vi "NI 5772 (AC) - DigitizerFIFOAvg (FPGA).vi"() -> ()   [LabVIEW 2020]
doc: "Example Description:\nThis example demonstrates how to enable Time Interleaved Sampling with the NI 5772 adapter module to achieve a sampling rate of 1.6GS/s. This example continuously acquires records of analog input data from the NI 5772 adapter module. It allows you to select an AI channel, trigger type, and record size. This VI must be compiled before it is run. \n\nRunning the VI:\nThis VI must be run from the NI 5772 - Getting Started (Host).vi. Refer to the host VI documentation for steps regarding running and configuring the FPGA VI. \n\nExecution Steps:\nRefer to the Block Diagram of this VI for execution comments."
uses:
  Controls/AI Trigger Type.ctl
  Controls/Aquire State.ctl
  <vilib>/Platform/TimedLoop/XDataNode/timing_clust.ctl
  <vilib>/Platform/TimedLoop/XDataNode/nitl_modes.ctl
  <vilib>/Platform/TimedLoop/XDataNode/wakeup.ctl
  Controls/DigitizerState.ctl
  <vilib>/rvi/Emulation/niFpgaGetClockAttributes.vi
  <vilib>/rvi/Emulation/niFpgaSctlEmulationGetInTimedLoop.vi
  <vilib>/rvi/Emulation/niFpgaEmulationReportErrorSimple.vi
  <vilib>/rvi/eio/common/nirviEmuTemplateMethod_errors.vi
  <vilib>/rvi/Emulation/niFpgaCriticalErrorInLSC.vi
  <vilib>/rvi/Emulation/niFpgaProcessEmulError.vi
  <vilib>/rvi/Emulation/niFpgaEmulationIsFPGAContextNoSignature.vi
  <vilib>/rvi/errors/niFpgaSetErrorForExecOnDevCompSimple.vi
  <vilib>/rvi/eio/common/nirviEmuReportErrorAndStop.vi
  <vilib>/rvi/DataTransferAndStorage/Container/Common/niFpgaContainerGetUniqueNameForEmu.vi
  <vilib>/rvi/FIFO/Fifo_Resource/nirvififoEmulationSetSize.vi
  <vilib>/rvi/FIFO/Fifo_Resource/nirviFifoEmulationQueueMgr.vi
  <instcachedir>/0/nirviFifoEmulationQueueMgr_E5CAEC123FF24DC58D834DCA3CDAA9B5.lvgen/nirviFifoEmulationQueueMgr_E5CAEC123FF24DC58D834DCA3CDAA9B5_004.vi
  <vilib>/Utility/error.llb/Clear Errors.vi
  <vilib>/rvi/FIFO/Fifo_Resource/nirvififoEmulationCreateLock.vi
  <vilib>/rvi/FIFO/Fifo_Resource/nirvififoEmulationObtainLock.vi
  <vilib>/rvi/FIFO/Fifo_Resource/nirvififoEmulationReleaseLock.vi
  <vilib>/rvi/occurrence/nirviWaitOnOccurrenceBase.vi
  <vilib>/rvi/errors/nirviReportUnexpectedCaseInternalError.vi
  <vilib>/rvi/errors/nirviReportUnexpectedCaseInternalError (U32).vi
  <instcachedir>/0/nirviFifoEmulationQueueMgr_E5CAEC123FF24DC58D834DCA3CDAA9B5.lvgen/nirviFifoEmulationQueueMgr_E5CAEC123FF24DC58D834DCA3CDAA9B5_008.vi
  <vilib>/rvi/FIFO/Fifo_Resource/nirvififoEmulationDetermineInputValidOut.vi
  <instcachedir>/0/nirviFifoEmulationQueueMgr_E5CAEC123FF24DC58D834DCA3CDAA9B5.lvgen/nirviFifoEmulationQueueMgr_E5CAEC123FF24DC58D834DCA3CDAA9B5_000.vi
  <vilib>/rvi/interface/RandomDataEmulation/niFpgaRandomDataHandleErrors.vi
  <instrlib>/_niInstr/Basic Elements/v1/FPGA/Private/Count Up U64.vi
  <vilib>/eio/EIONode/EIONode.xnode
  <vilib>/rvi/DataTransferAndStorage/Container/XNode/niFpgaContainer.xnode
  <vilib>/rvi/FIFO/Fifo_Resource/nirvififoEmulationRead.vi
  <vilib>/Platform/TimedLoop/XDataNode/XDataNode.xnode
  <vilib>/rvi/FIFO/Fifo_Resource/nirvififoEmulationGetNumberOfElementsToRead.vi
  <vilib>/rvi/FIFO/Fifo_Resource/nirvififoEmulationWrite.vi
  <vilib>/rvi/interface/RandomDataEmulation/nirviRandomDataFpgaReadWriteTemplate.vi
  <vilib>/Platform/TimedLoop/XDataNode/XDNodeRunTimeDep.lvlib
  <instrlib>/_niInstr/Basic Elements/v1/FPGA/niInstr Basic Elements v1 FPGA.lvlib
  <vilib>/rvi/Memory/Memory_Emulation/nirvimemoryFastEmulation.vi
  <vilib>/rvi/Memory/Memory_Emulation/nirvimemoryEmulation.vi
panel:
  out "DMA FIFO Overflow? 2":bool caption="FIFO Overflow?"
  out "WaitForWave\nCompletion":u16
  in  "Wave Sampling Rate":sgl
  in  "WaveSampleCount":sgl format="%#_13g"
  in  "Delay (us)":sgl
  in  "AvgCount_powerOf2":i16=1
  out "DMA FIFO Overflow?":bool caption="FIFO Overflow?"
  out "Removed\nElement":u64
  out "AvgCount":u16=1
  in  "vi/nGenTrig":bool
  in  "TrigIn Simulate":bool
  out "Trig Count":u64
  in  "Clear Count":bool
  out "Delay after Trig [cycles]":u16
  out "TS FIFO In Overflow?":bool caption="FIFO Overflow?"
  in  "Samples Per Trigger":u16=512 min=1 step=1
  in  "Arm Trigger":bool
  in  "User Command Commit":bool
  in  "User Command":u8
  out "User Command Idle":bool
  out "User Command Status":u8
  in  "User Data 0":u16
  in  "User Data 1":u8
  out "PLL Locked":bool
  out "User Error":bool
  out "Configured?":bool
  in  "Trigger Level":i16
  in  "Trigger Type":T1
  # "Resource Configuration"
  # "Analog Input"
  # "Clock Configuration"
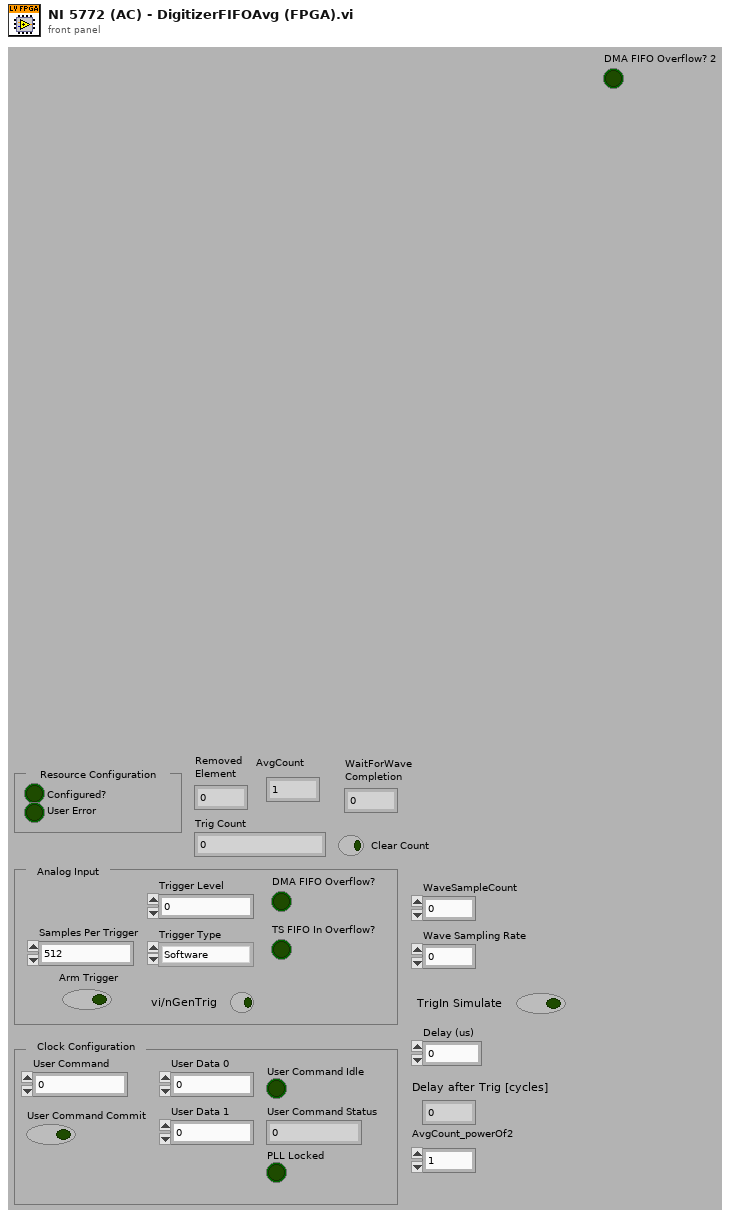
[diagram p1: front panel]
types:
  T1 = typedef "AI Trigger Type.ctl" = enum8{"Software", "Data Edge"}
  T2 = typedef "DigitizerState.ctl" = enum16{"Init", "Build/Clear Accumulator", "GetData", "AverageCountCheck", "SendtoHost"}
  T3 = typedef "Aquire State.ctl" = enum8{"Idle", "Wait for Trigger", "AlignWave", "Hold Aquire", "Acquire", "WaitForWaveCompletion", "CheckAvg"}
  T4 = typedef "XDNodeRunTimeDep.lvlib/timing_clust.ctl" = cluster{"Expected End [f-1]":u64, "Actual End [f-1]":u64, "Finished Late? [f-1]":bool, "Expected End [i-1]":u64, "Actual End [i-1]":u64, "Finished Late? [i-1]":bool, "Expected Start [i]":u64, "Actual Start [i]":u64, "Expected Start [f]":u64, "Actual Start [f]":u64, "Source Name":string, "Structure Name":string, "Period":i64, "Deadline":i64, "Offset":i64, "Start":i64, "Priority":i32, "Timeout":i32, "Mode":T5, "Wakeup Reason":T6, "Error":errorcluster, "Source Type":string, "Secondary Source Type":string, "Global End Time":u64, "Global Start Time":u64, "Frame Duration":u64, "Iteration Duration":u64, "Assigned CPU":i32, "I/O Scan Engine Mode":u32}
  T5 = typedef "XDNodeRunTimeDep.lvlib/nitl_modes.ctl" = enum32{"No Change", "Process missed periods, maintain original phase", "Discard missed periods, maintain original phase", "Process missed periods, ignore original phase", "Discard missed periods, ignore original phase"}
  T6 = typedef "XDNodeRunTimeDep.lvlib/wakeup.ctl" = enum32{"Normal", "Aborted", "Asynchronous wakeup", "Timing source error", "Timed loop error", "Timeout"}
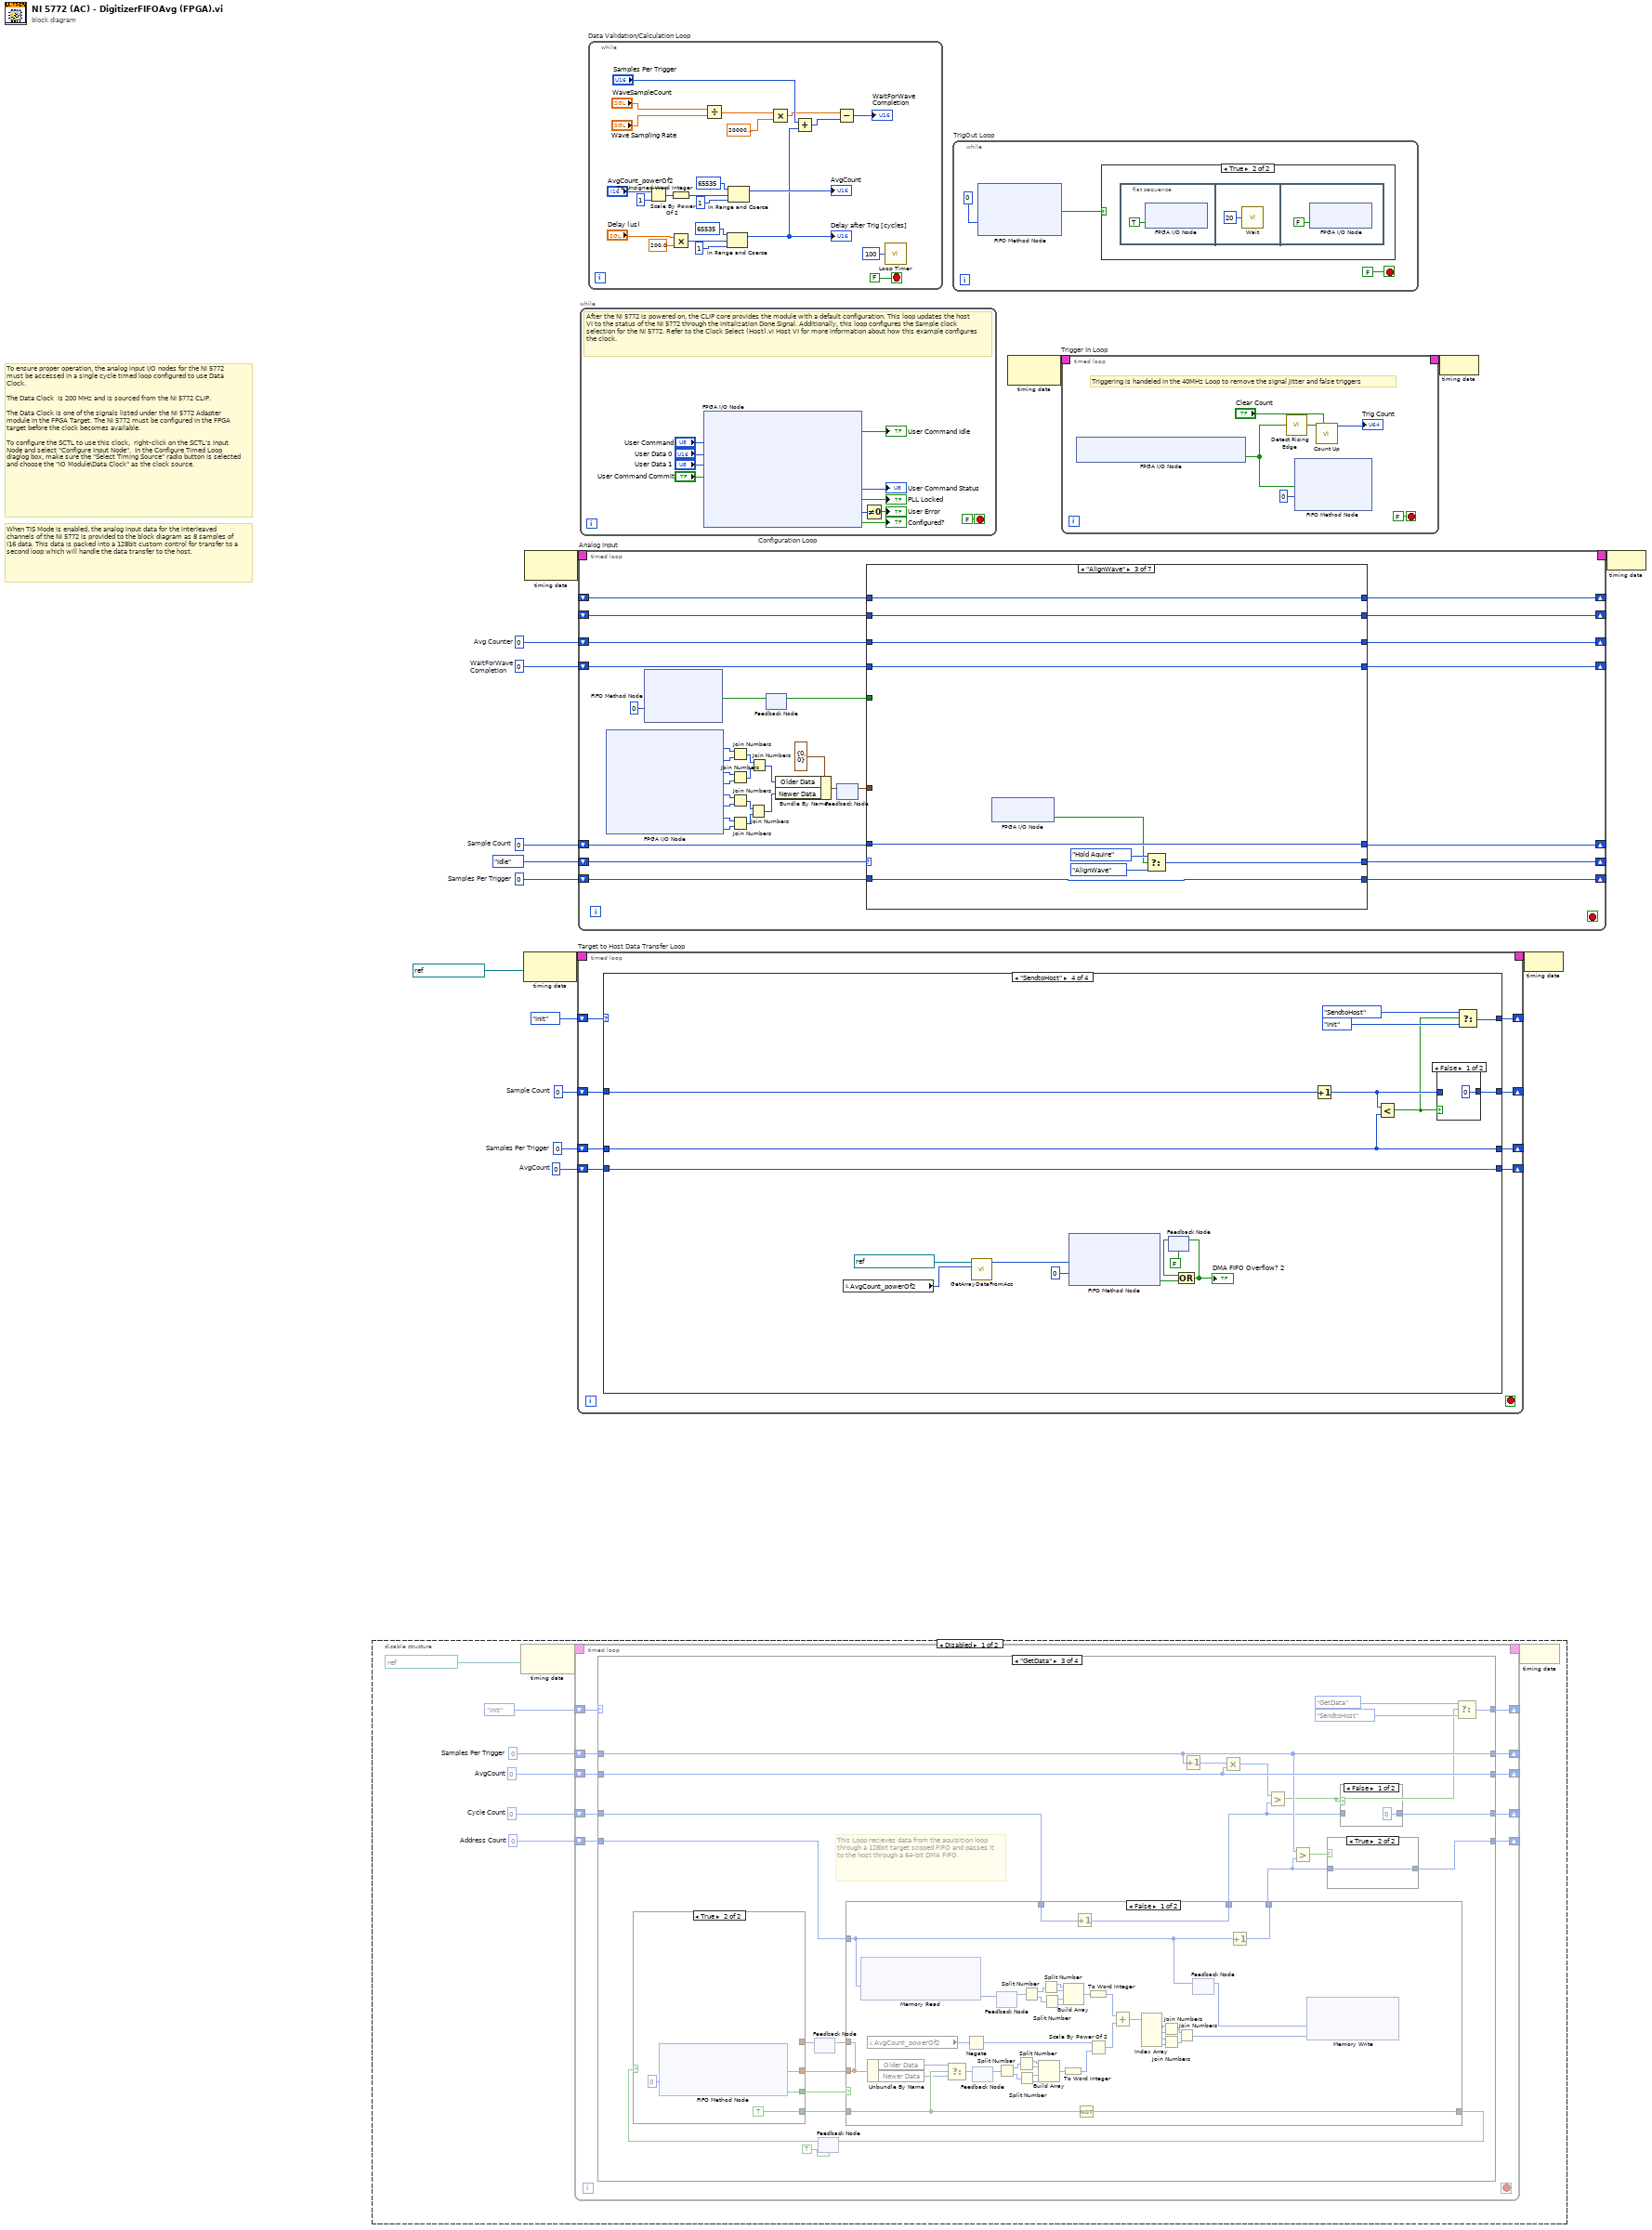
[diagram p0: block diagram]
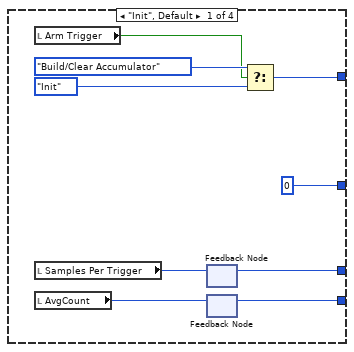
[diagram p2: hidden frame]
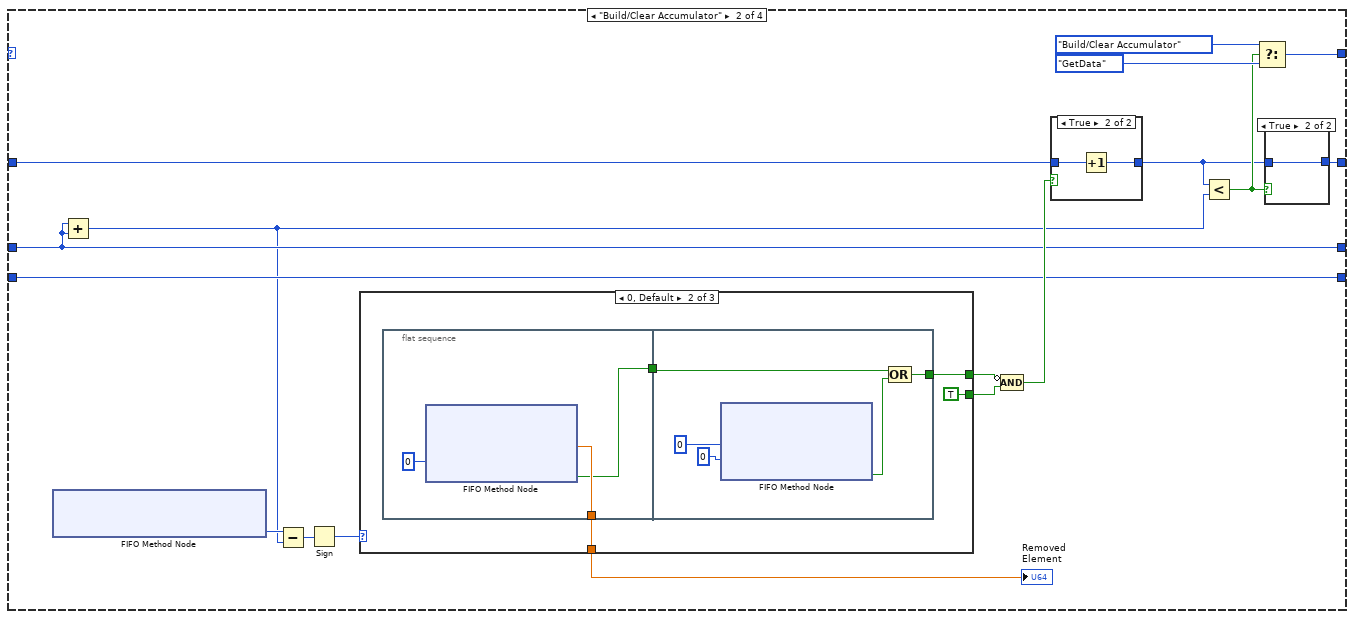
[diagram p3: hidden frame]
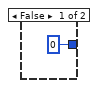
[diagram p4: hidden frame]
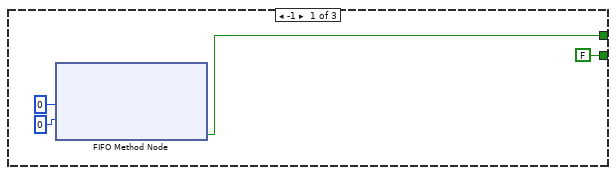
[diagram p6: hidden frame]
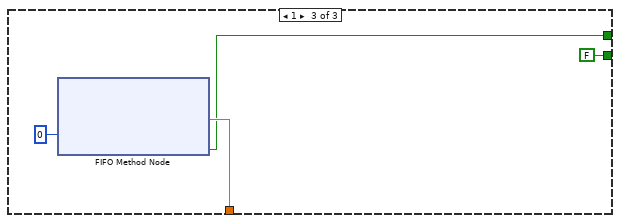
[diagram p7: hidden frame]
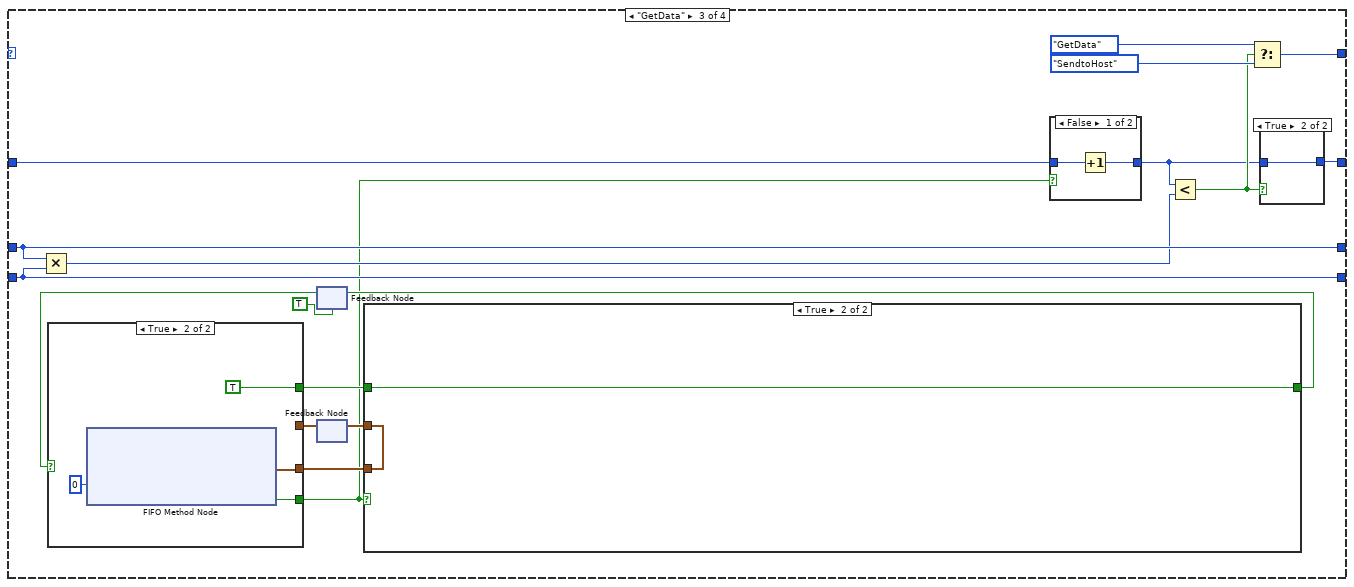
[diagram p8: hidden frame]
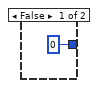
[diagram p9: hidden frame]
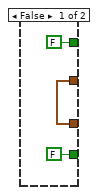
[diagram p11: hidden frame]
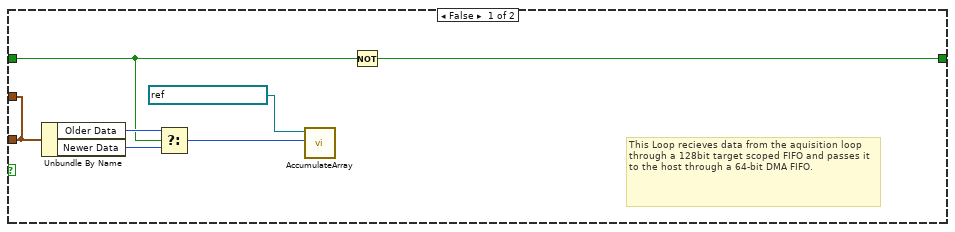
[diagram p12: hidden frame]
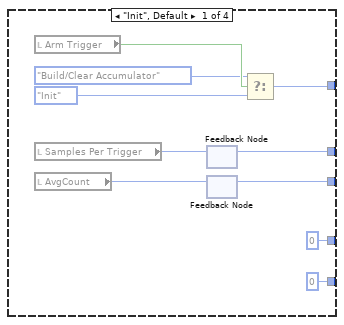
[diagram p14: hidden frame]
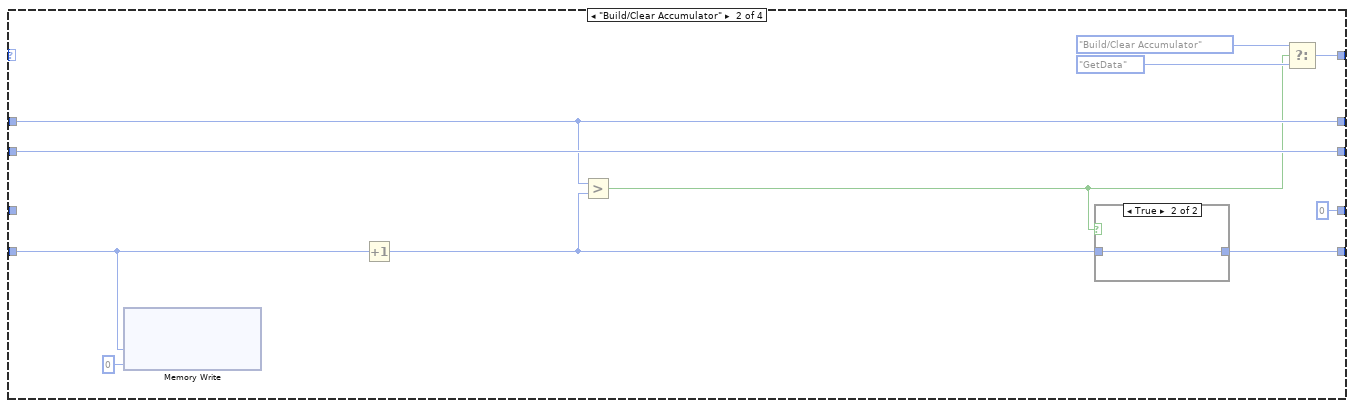
[diagram p15: hidden frame]
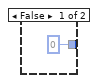
[diagram p16: hidden frame]
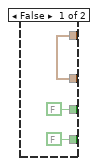
[diagram p18: hidden frame]
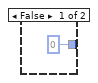
[diagram p20: hidden frame]
diagram:
  w1 = u16 0  # Sample Count
  w2 = u16 0  # Samples Per Trigger
  w3 = u16 0  # AvgCount
  w8 = u16 0  # WaitForWave Completion
  w9 = u16 0  # Avg Counter
  w12 = u16 0  # Samples Per Trigger
  w13 = u16 0  # Sample Count
  # "When TIS Mode is enabled, the analog input data for the interleaved channels of the NI 5772 is provided to the block diagram as 8 samples of I16 data. This data is packed into a 128bit custom control for transfer to a second loop which will handle the data transfer to the host."
  # "To ensure proper operation, the analog input I/O nodes for the NI 5772 must be accessed in a single cycle timed loop configured to use Data Clock. \n\nThe Data Clock  is 200 MHz and is sourced from the NI 5772 CLIP.\n\nThe Data Clock is one of the signals listed under the NI 5772 Adapter module in the FPGA Target. The NI 5772 must be configured in the FPGA target before the clock becomes available. \n\nTo configure the SCTL to use this clock,  right-click on the SCTL's Input Node and select \"Configure Input Node\".  In the Configure Timed Loop diaglog box, make sure the \"Select Timing Source\" radio button is selected and choose the \"IO Module\\Data Clock\" as the clock source."
  n1 = disable-structure shown="Disabled" {
    frame Disabled {
      w17 = u32 0  # Cycle Count
      w18 = u32 0  # Address Count
      w19 = u16 0  # AvgCount
      w20 = u16 0  # Samples Per Trigger
      n2 = node-c288(refnum<k21> "100 MHz Clock" ("Source Name")) -> (w24:T4)
      n3 = timed-loop {
        timing: w24 -> [_]
        timing-out: [_] -> w23
        shift-right: [w33] -> _
        shift-left: DigitizerState."Init" -> [w34]
        shift-right: [w32] -> _
        shift-left: w20 -> [w30]
        shift-right: [w31] -> _
        shift-left: w19 -> [w29]
        shift-right: [w27] -> _
        shift-left: w18 -> [w28]
        shift-right: [w25] -> _
        shift-left: w17 -> [w26]
        stop <- _ stop-if-true
        n4 = case shown="\"GetData\"" w34 {
          tunnel: [w39 w49 w78 w150] -> w33
          tunnel: [w38 w52 w62 w140] -> w32
          tunnel: [w37 w53 w68 w153] -> w31
          tunnel: w30 -> [_ w52 w62 w140]
          tunnel: w29 -> [_ w53 w68 w153]
          tunnel: w28 -> [_ w55 w65 w142]
          tunnel: [u32 0 w46 w77 w148] -> w27
          tunnel: w26 -> [_ _ w61 w137]
          tunnel: [u32 0 ("Cycle Count") u32 0 ("Cycle Count") w58 w138] -> w25
          frame "Init", Default {
            n5 = local read "Arm Trigger"() -> (w44:bool)
            n6 = local read "Samples Per Trigger"() -> (w40:u16)
            n7 = local read "AvgCount"() -> (w41:u16)
            n8 = feedback #1() -> (w38:u16)  [unwired: 1 in]
            n9 = feedback-in #1(w40) -> ()
            n10 = feedback #2() -> (w37:u16)  [unwired: 1 in]
            n11 = feedback-in #2(w41) -> ()
            n12 = Select(t=DigitizerState."Build/Clear Accumulator", s=w44, f=DigitizerState."Init") -> (s? t:f=w39:T2)
          }
          frame "Build/Clear Accumulator" {
            n13 = xnode ("Memory Write")("Address"=w55, "Data"=u64 0) -> ()  [unwired: 1 in, 1 out]
            n14 = Increment(x=w55) -> (x+1=w47:u32)
            n15 = Greater?(x=w52, y=w47) -> (0:w48:bool)
            n16 = case shown="True" w48 {
              tunnel: w47 -> [_ w57]
              tunnel: [u32 0 w57] -> w46
              frame False {
              }
              frame True {
              }
            }
            n17 = Select(t=DigitizerState."Build/Clear Accumulator", s=w48, f=DigitizerState."GetData") -> (s? t:f=w49:T2)
          }
          frame "GetData" {
            # "This Loop recieves data from the aquisition loop through a 128bit target scoped FIFO and passes it to the host through a 64-bit DMA FIFO."
            n18 = feedback #3() -> (w72:cluster{"Older Data":u64, "Newer Data":u64})  [unwired: 1 in]
            n19 = feedback #4(TRUE ("Timed Out?")) -> (w71:bool)
            n20 = case shown="True" w71 {
              tunnel: [w83 w86] -> w74
              tunnel: [FALSE ("Timed Out?") w87] -> w76
              tunnel: [FALSE ("Timed Out?") TRUE ("Timed Out?")] -> w75
              tunnel: w72 -> [w83 _]
              frame False {
              }
              frame True {
                n21 = xnode ("FIFO Method Node")("Timeout"=0) -> ("Element"=w86:cluster{"Older Data":u64, "Newer Data":u64}, "Timed Out?"=w87:bool)  [unwired: 1 in, 1 out]
              }
            }
            n22 = case shown="False" w76 {
              tunnel: [w128 w134] -> w70
              tunnel: w75 -> [w129 w134]
              tunnel: w74 -> [w127 w133]
              tunnel: [w127 w133] -> w73
              tunnel: w65 -> [w104 w132]
              tunnel: [w117 w132] -> w64
              tunnel: w61 -> [w93 w131]
              tunnel: [w92 w131] -> w59
              frame False {
                n23 = xnode ("Memory Read")("Address"=w104) -> ("Data"=w95:u64)  [unwired: 1 in, 1 out]
                n24 = local read "AvgCount_powerOf2"() -> (w108:i16)
                n25 = Unbundle By Name(w127) -> ("Older Data"=w130:u64, "Newer Data"=w126:u64)
                n26 = Select(t=w130, s=w129, f=w126) -> (s? t:f=w118:u64)
                n27 = Negate(x=w108) -> (-x=w109:i16)
                n28 = feedback-in #5(w118) -> ()
                n29 = feedback #5() -> (w91:u64)  [unwired: 1 in]
                n30 = feedback-in #6(w95) -> ()
                n31 = feedback #6() -> (w94:u64)  [unwired: 1 in]
                n32 = Split Number(x=w91) -> (hi(x)=w120:u32, lo(x)=w121:u32)
                n33 = Split Number(x=w120) -> (hi(x)=w122:u16, lo(x)=w123:u16)
                n34 = Split Number(x=w121) -> (hi(x)=w124:u16, lo(x)=w125:u16)
                n35 = Split Number(x=w94) -> (hi(x)=w116:u32, lo(x)=w115:u32)
                n36 = Build Array(w122, w123, w124, w125) -> (w119:u16[])
                n37 = Split Number(x=w116) -> (hi(x)=w114:u16, lo(x)=w113:u16)
                n38 = Split Number(x=w115) -> (hi(x)=w112:u16, lo(x)=w111:u16)
                n39 = To Word Integer(number=w119) -> (16bit integer=w107:i16[])
                n40 = Build Array(w114, w113, w112, w111) -> (w110:u16[])
                n41 = Increment(x=w93) -> (x+1=w92:u32)
                n42 = Not(x=w129) -> (.not. x?=w128:bool)
                n43 = To Word Integer(number=w110) -> (16bit integer=w105:i16[])
                n44 = Scale By Power Of 2(n=w109, x=w107) -> (x*2^n=w106:i16[])
                n45 = Add(x=w105, y=w106) -> (x+y=w97:i16[])
                n46 = Index Array(array=w97) -> (element #1=w100:i16, element #2=w101:i16, element #3=w102:i16, element #4=w103:i16)  [unwired: 4 in]
                n47 = Join Numbers(hi=w100, lo=w101) -> ((hi.lo)=w98:u32)
                n48 = Join Numbers(hi=w102, lo=w103) -> ((hi.lo)=w99:u32)
                n49 = Join Numbers(hi=w98, lo=w99) -> ((hi.lo)=w96:u64)
                n50 = feedback-in #7(w104) -> ()
                n51 = feedback #7() -> (w90:u32)  [unwired: 1 in]
                n52 = Increment(x=w104) -> (x+1=w117:u32)
                n53 = xnode ("Memory Write")("Address"=w90, "Data"=w96) -> ()  [unwired: 1 in, 1 out]
              }
              frame True {
              }
            }
            n54 = feedback-in #3(w73) -> ()
            n55 = feedback-in #4(w70) -> ()
            n56 = Increment(x=w62) -> (x+1=w63:u16)
            n57 = Multiply(x=w63, y=w68) -> (x*y=w67:u16)
            n58 = Greater?(x=w67, y=w59) -> (0:w60:bool)
            n59 = Greater?(x=w62, y=w64) -> (0:w66:bool)
            n60 = case shown="True" w66 {
              tunnel: w64 -> [_ w136]
              tunnel: [u32 0 w136] -> w77
              frame False {
              }
              frame True {
              }
            }
            n61 = case shown="False" w60 {
              tunnel: w59 -> [_ w82]
              tunnel: [u32 0 ("Cycle Count") w82] -> w58
              frame False {
              }
              frame True {
              }
            }
            n62 = Select(t=DigitizerState."GetData", s=w60, f=DigitizerState."SendtoHost") -> (s? t:f=w78:T2)
          }
          frame "SendtoHost" {
            n63 = feedback-in #8(w142) -> ()
            n64 = feedback #8() -> (w144:u32)  [unwired: 1 in]
            n65 = Increment(x=w142) -> (x+1=w139:u32)
            n66 = xnode ("Memory Read")("Address"=w144) -> ("Data"=w147:u64)  [unwired: 1 in, 1 out]
            n67 = feedback-in #9(w147) -> ()
            n68 = feedback #9() -> (w146:u64)  [unwired: 1 in]
            n69 = Greater Than 0?(x=w137) -> (x > 0?=w143:bool)
            n70 = case shown="True" w143 {
              tunnel: w146 -> [_ w154]
              frame False {
              }
              frame True {
                # "Monitor for any DMA FIFO timeouts"
                n71 = xnode ("FIFO Method Node")("Element"=w154, "Timeout"=0) -> ("Timed Out?"=w158:bool)  [unwired: 1 in, 1 out]
                n72 = feedback #10(FALSE) -> (w157:bool)
                n73 = Compound Arithmetic op=OR(w157, w158) -> (w159:bool)
                "DMA FIFO Overflow?" <- w159
                n74 = feedback-in #10(w159) -> ()
              }
            }
            n75 = Increment(x=w137) -> (x+1=w138:u32)
            n76 = Increment(x=w140) -> (x+1=w145:u16)
            n77 = Greater?(x=w145, y=w138) -> (0:w149:bool)
            n78 = Greater?(x=w140, y=w139) -> (0:w141:bool)
            n79 = case shown="False" w141 {
              tunnel: w139 -> [_ w161]
              tunnel: [u32 0 w161] -> w148
              frame False {
              }
              frame True {
              }
            }
            n80 = Select(t=DigitizerState."SendtoHost", s=w149, f=DigitizerState."Init") -> (s? t:f=w150:T2)
          }
        }
      }
      n81 = node-c288(w23) -> ()
    }
    frame Enabled {
    }
  }
  n82 = node-c288(refnum<k21> "100 MHz Clock" ("Source Name")) -> (w7:T4)
  n83 = node-c288() -> (w16:T4)  [unwired: 1 in]
  n84 = timed-loop "Target to Host Data Transfer Loop" {
    timing: w7 -> [_]
    timing-out: [_] -> w6
    shift-right: [w170] -> _
    shift-left: DigitizerState."Init" -> [w175]
    shift-right: [w174] -> _
    shift-left: w2 -> [w173]
    shift-right: [w172] -> _
    shift-left: w3 -> [w171]
    shift-right: [w168] -> _
    shift-left: w1 -> [w169]
    stop <- _ stop-if-true
    n85 = case shown="\"SendtoHost\"" w175 {
      tunnel: [w183 w186 w237 w274] -> w174
      tunnel: w173 -> [_ w186 w237 w274]
      tunnel: [w181 w190 w236 w282] -> w172
      tunnel: w171 -> [_ w190 w236 w282]
      tunnel: [w177 w197 w231 w279] -> w170
      tunnel: w169 -> [_ w192 w230 w277]
      tunnel: [u16 0 ("Sample Count") w188 w229 w275] -> w168
      frame "Init", Default {
        n86 = local read "Arm Trigger"() -> (w178:bool)
        n87 = local read "Samples Per Trigger"() -> (w184:u16)
        n88 = local read "AvgCount"() -> (w182:u16)
        n89 = feedback #11() -> (w183:u16)  [unwired: 1 in]
        n90 = feedback-in #11(w184) -> ()
        n91 = feedback #12() -> (w181:u16)  [unwired: 1 in]
        n92 = feedback-in #12(w182) -> ()
        n93 = Select(t=DigitizerState."Build/Clear Accumulator", s=w178, f=DigitizerState."Init") -> (s? t:f=w177:T2)
      }
      frame "Build/Clear Accumulator" {
        n94 = xnode ("FIFO Method Node")() -> ("Number of Elements to Read"=w201:u32)  [unwired: 1 in, 1 out]
        n95 = Add(x=w186, y=w186) -> (x+y=w185:u16)
        n96 = Subtract(x=w201, y=w185) -> (x-y=w200:i8)
        n97 = Sign(1:w200) -> (0:w199:i8)
        n98 = case shown="0, Default" w199 {
          tunnel: [_ w214 w225] -> w198
          tunnel: [w208 w212 w224] -> w194
          tunnel: [FALSE TRUE FALSE] -> w193
          frame -1 {
            n99 = xnode ("FIFO Method Node")("Element"=u64 0, "Timeout"=0) -> ("Timed Out?"=w208:bool)  [unwired: 1 in, 1 out]
          }
          frame 0, Default {
            n100 = flat-sequence {
              tunnel: [w216] -> w214
              tunnel: [w215] -> w213
              tunnel: w213 -> [w220]
              tunnel: [w218] -> w212
              frame #0 {
                n101 = xnode ("FIFO Method Node")("Timeout"=0) -> ("Element"=w216:sgl, "Timed Out?"=w215:bool)  [unwired: 1 in, 1 out]
              }
              frame #1 {
                n102 = xnode ("FIFO Method Node")("Element"=u64 0 ("y"), "Timeout"=0) -> ("Timed Out?"=w219:bool)  [unwired: 1 in, 1 out]
                n103 = Compound Arithmetic op=OR(w220, w219) -> (w218:bool)
              }
            }
          }
          frame 1 {
            n104 = xnode ("FIFO Method Node")("Timeout"=0) -> ("Element"=w225:sgl, "Timed Out?"=w224:bool)  [unwired: 1 in, 1 out]
          }
        }
        "Removed\nElement" <- w198
        n105 = Compound Arithmetic op=AND(invert w194, w193) -> (w191:bool)
        n106 = case shown="True" w191 {
          tunnel: w192 -> [w204 w206]
          tunnel: [w204 w205] -> w187
          frame False {
          }
          frame True {
            n107 = Increment(x=w206) -> (x+1=w205:u16)
          }
        }
        n108 = Less?(x=w187, y=w185) -> (x < y?=w189:bool)
        n109 = Select(t=DigitizerState."Build/Clear Accumulator", s=w189, f=DigitizerState."GetData") -> (s? t:f=w197:T2)
        n110 = case shown="True" w189 {
          tunnel: [u16 0 ("Sample Count") w203] -> w188
          tunnel: w187 -> [_ w203]
          frame False {
          }
          frame True {
          }
        }
      }
      frame "GetData" {
        n111 = Multiply(x=w237, y=w236) -> (x*y=w228:u16)
        n112 = feedback #13(TRUE ("Timed Out?")) -> (w242:bool)
        n113 = feedback #14() -> (w241:cluster{"Older Data":u64, "Newer Data":u64})  [unwired: 1 in]
        n114 = case shown="True" w242 {
          tunnel: [w250 w253] -> w239
          tunnel: [FALSE ("Timed Out?") w254] -> w227
          tunnel: [FALSE ("Timed Out?") TRUE ("Timed Out?")] -> w238
          tunnel: w241 -> [w250 _]
          frame False {
          }
          frame True {
            n115 = xnode ("FIFO Method Node")("Timeout"=0) -> ("Element"=w253:cluster{"Older Data":u64, "Newer Data":u64}, "Timed Out?"=w254:bool)  [unwired: 1 in, 1 out]
          }
        }
        n116 = case shown="True" w227 {
          tunnel: [w261 w265] -> w243
          tunnel: w238 -> [w262 w265]
          tunnel: w239 -> [w260 w264]
          tunnel: [w260 w264] -> w240
          frame False {
            # "This Loop recieves data from the aquisition loop through a 128bit target scoped FIFO and passes it to the host through a 64-bit DMA FIFO."
            n117 = Unbundle By Name(w260) -> ("Older Data"=w263:u64, "Newer Data"=w259:u64)
            n118 = Select(t=w263, s=w262, f=w259) -> (s? t:f=w257:u64)
            n119 = call "AccumulateArray.vi"("Timeout"=w257, "Refnum in"=refnum<k21> "AveragingFIFO-A" ("FIFO In")) -> ()  [unwired: 10 in]
            n120 = Not(x=w262) -> (.not. x?=w261:bool)
          }
          frame True {
          }
        }
        n121 = feedback-in #13(w243) -> ()
        n122 = feedback-in #14(w240) -> ()
        n123 = case shown="False" w227 {
          tunnel: w230 -> [w248 w249]
          tunnel: [w247 w249] -> w232
          frame False {
            n124 = Increment(x=w248) -> (x+1=w247:u16)
          }
          frame True {
          }
        }
        n125 = Less?(x=w232, y=w228) -> (x < y?=w233:bool)
        n126 = Select(t=DigitizerState."GetData", s=w233, f=DigitizerState."SendtoHost") -> (s? t:f=w231:T2)
        n127 = case shown="True" w233 {
          tunnel: [u16 0 ("Sample Count") w246] -> w229
          tunnel: w232 -> [_ w246]
          frame False {
          }
          frame True {
          }
        }
      }
      frame "SendtoHost" {
        n128 = local read "AvgCount_powerOf2"() -> (w273:i16)
        n129 = call "GetArrayDataFromAcc.vi"("AvgCount_powerOf2"=w273, "Refnum in"=refnum<k21> "AveragingFIFO-A" ("FIFO In")) -> ("Numeric"=w271:u64)  [unwired: 9 in]
        n130 = xnode ("FIFO Method Node")("Element"=w271, "Timeout"=0) -> ("Timed Out?"=w267:bool)  [unwired: 1 in, 1 out]
        n131 = feedback #15(FALSE) -> (w268:bool)
        n132 = Compound Arithmetic op=OR(w268, w267) -> (w266:bool)
        "DMA FIFO Overflow? 2" <- w266
        n133 = feedback-in #15(w266) -> ()
        n134 = Increment(x=w277) -> (x+1=w278:u16)
        n135 = Less?(x=w278, y=w274) -> (x < y?=w276:bool)
        n136 = case shown="False" w276 {
          tunnel: [u16 0 ("Sample Count") w284] -> w275
          tunnel: w278 -> [_ w284]
          frame False {
          }
          frame True {
          }
        }
        n137 = Select(t=DigitizerState."SendtoHost", s=w276, f=DigitizerState."Init") -> (s? t:f=w279:T2)
      }
    }
  }
  n138 = timed-loop "Analog Input" {
    timing: w16 -> [_]
    timing-out: [_] -> w15
    shift-right: [w319] -> _
    shift-left: Aquire_State."Idle" ("Acquire State") -> [w309]
    shift-right: [w320] -> _
    shift-left: w13 -> [w310]
    shift-right: [w318] -> _
    shift-left: w12 -> [w308]
    shift-right: [w295] -> _
    shift-left: _ -> [w294]
    shift-right: [w293] -> _
    shift-left: _ -> [w292]
    shift-right: [w290] -> _
    shift-left: w9 -> [w291]
    shift-right: [w288] -> _
    shift-left: w8 -> [w287]
    stop <- _ stop-if-true
    n139 = xnode "FPGA I/O Node"() -> ("IO Module\\AI 1 Data N-3"=w301:i16, "IO Module\\AI 0 Data N-3"=w300:i16, "IO Module\\AI 1 Data N-2"=w299:i16, "IO Module\\AI 0 Data N-2"=w298:i16, "IO Module\\AI 1 Data N-1"=w302:i16, "IO Module\\AI 0 Data N-1"=w303:i16, "IO Module\\AI 1 Data N"=w304:i16, "IO Module\\AI 0 Data N"=w305:i16)  [unwired: 8 in, 8 out]
    n140 = xnode ("FIFO Method Node")("Timeout"=0) -> ("Element"=w296:bool)  [unwired: 1 in, 2 out]
    n141 = Join Numbers(hi=w301, lo=w300) -> ((hi.lo)=w313:u32)
    n142 = Join Numbers(hi=w299, lo=w298) -> ((hi.lo)=w315:u32)
    n143 = Join Numbers(hi=w302, lo=w303) -> ((hi.lo)=w314:u32)
    n144 = Join Numbers(hi=w304, lo=w305) -> ((hi.lo)=w316:u32)
    n145 = Join Numbers(hi=w314, lo=w316) -> ((hi.lo)=w306:u64)
    n146 = Join Numbers(hi=w313, lo=w315) -> ((hi.lo)=w307:u64)
    n147 = feedback-in #16(w296) -> ()
    n148 = feedback #16() -> (w289:bool)  [unwired: 1 in]
    n149 = Bundle By Name(cluster=cluster{"Older Data":u64, "Newer Data":u64} {"Older Data"=0, "Newer Data"=0} ("Element"), "Older Data"=w307, "Newer Data"=w306) -> (w311:cluster{"Older Data":u64, "Newer Data":u64})
    n150 = feedback #17() -> (w317:cluster{"Older Data":u64, "Newer Data":u64})  [unwired: 1 in]
    n151 = feedback-in #17(w311) -> ()
    n152 = case shown="\"AlignWave\"" w309 {
      tunnel: [u16 0 u16 0 w373 w385 w394 w416 u16 0] -> w320
      tunnel: w310 -> [_ _ w373 w384 w409 w418 _]
      tunnel: [w332 w344 w376 w388 w408 w421 w432] -> w319
      tunnel: [w329 w348 w374 w386 w405 w419 w430] -> w318
      tunnel: w308 -> [_ w348 w374 w386 w405 w419 w430]
      tunnel: w317 -> [_ w347 _ _ w404 _ _]
      tunnel: w289 -> [_ w342 _ _ _ _ _]
      tunnel: [w327 w340 w372 w383 w398 w417 w429] -> w295
      tunnel: w294 -> [_ w340 w372 w383 w398 w417 w429]
      tunnel: [w325 w339 w371 w381 w397 w414 w427] -> w293
      tunnel: w292 -> [_ w339 w371 w381 w397 w414 w427]
      tunnel: [u16 0 ("Avg Count") w338 w370 w380 w396 w413 w426] -> w290
      tunnel: w291 -> [_ w338 w370 w380 w396 w413 w428]
      tunnel: [w321 w336 w368 w378 w392 w412 w423] -> w288
      tunnel: w287 -> [_ w336 w368 w378 w392 w412 w423]
      frame "Idle", Default {
        # "This state will wait for the host VI to arm the trigger."
        n153 = feedback-in #18("Arm Trigger") -> ()
        n154 = feedback #18() -> (w330:bool)  [unwired: 1 in]
        n155 = local read "WaitForWave\nCompletion"() -> (w322:u16)
        n156 = Select(t=Aquire_State."Wait for Trigger" ("Acquire State"), s=w330, f=Aquire_State."Idle" ("Acquire State")) -> (s? t:f=w332:T3)
        n157 = local read "Delay after Trig [cycles]"() -> (w328:u16)
        n158 = local read "AvgCount"() -> (w326:u16)
        n159 = local read "Samples Per Trigger"() -> (w323:u16)
        n160 = feedback #19() -> (w327:u16)  [unwired: 1 in]
        n161 = feedback-in #19(w328) -> ()
        n162 = feedback #20() -> (w325:u16)  [unwired: 1 in]
        n163 = feedback-in #20(w326) -> ()
        n164 = feedback #21() -> (w321:u16)  [unwired: 1 in]
        n165 = feedback-in #21(w322) -> ()
        n166 = feedback-in #22(w323) -> ()
        n167 = feedback #22() -> (w329:u16)  [unwired: 1 in]
      }
      frame "Wait for Trigger" {
        # "After the trigger is armed, this state monitors for the specific trigger condition to begin the acquisition."
        n168 = feedback-in #23("Trigger Type") -> ()
        n169 = feedback #23() -> (w341:T1)  [unwired: 1 in]
        n170 = case shown="\"Software\", Default" w341 {
          tunnel: w347 -> [_ w367]
          tunnel: [w358 w359] -> w337
          tunnel: w342 -> [w353 _]
          frame "Software", Default {
            n171 = Compound Arithmetic op=AND(w353, invert "vi/nGenTrig") -> (w357:bool)
            n172 = Compound Arithmetic op=AND("vi/nGenTrig", "TrigIn Simulate") -> (w355:bool)
            n173 = Compound Arithmetic op=OR(w357, w355) -> (w352:bool)
            n174 = call <instrlib>:"Detect Rising Edge.vi"("signal"=w352) -> ("edge detected"=w358:bool)  [unwired: 14 in]
          }
          frame "Data Edge" {
            # "Begins the acquisition after the analog input rises above the trigger level."
            n175 = Unbundle By Name(w367) -> ("Older Data"=w365:u64, "Newer Data"=w363:u64)
            n176 = feedback-in #24("Trigger Level") -> ()
            n177 = feedback #24() -> (w361:i16)  [unwired: 1 in]
            n178 = feedback-in #25(w365) -> ()
            n179 = feedback #25() -> (w360:u64)  [unwired: 1 in]
            n180 = feedback-in #26(w363) -> ()
            n181 = feedback #26() -> (w362:u64)  [unwired: 1 in]
            n182 = call "Data Edge Trigger 8 Samples.vi"("Trigger Level"=w361, "Newer Data In"=w362, "Older Data In"=w360) -> ("Trigger"=w366:bool)  [unwired: 8 in]
            n183 = feedback-in #27(w366) -> ()
            n184 = feedback #27() -> (w359:bool)  [unwired: 1 in]
          }
        }
        n185 = case shown="True" w337 {
          selector: w337 -> [_ w351]
          frame False {
          }
          frame True {
            n186 = xnode ("FIFO Method Node")("Element"=w351, "Timeout"=0) -> ()  [unwired: 1 in, 2 out]
          }
        }
        n187 = Select(t=Aquire_State."AlignWave" ("Acquire State"), s=w337, f=Aquire_State."Wait for Trigger") -> (s? t:f=w344:T3)
      }
      frame "AlignWave" {
        n188 = xnode "FPGA I/O Node"() -> ("PXI_Trig0"=w369:bool)  [unwired: 1 in, 1 out]
        n189 = Select(t=Aquire_State."Hold Aquire" ("Acquire State"), s=w369, f=Aquire_State."AlignWave" ("Acquire State")) -> (s? t:f=w376:T3)
      }
      frame "Hold Aquire" {
        n190 = Increment(x=w384) -> (x+1=w382:u16)
        n191 = Greater?(x=w383, y=w382) -> (0:w379:bool)
        n192 = Select(t=Aquire_State."Hold Aquire" ("Acquire State"), s=w379, f=Aquire_State."Acquire" ("Acquire State")) -> (s? t:f=w388:T3)
        n193 = case shown="True" w379 {
          tunnel: [u16 0 w391] -> w385
          tunnel: w382 -> [_ w391]
          frame False {
          }
          frame True {
          }
        }
      }
      frame "Acquire" {
        # "Monitor for any  FIFO timeouts"
        # "While in this state, data is pushed into a DMA FIFO until the desired number of samples per record have been acquired."
        n194 = xnode ("FIFO Method Node")("Element"=w404, "Timeout"=0) -> ("Timed Out?"=w399:bool)  [unwired: 1 in, 1 out]
        n195 = Increment(x=w409) -> (x+1=w395:u16)
        n196 = Less?(x=w395, y=w405) -> (x < y?=w393:bool)
        n197 = feedback #28(FALSE) -> (w400:bool)
        n198 = Or(x=w400, y=w399) -> (x .or. y?=w401:bool)
        "TS FIFO In Overflow?" <- w401
        n199 = feedback-in #28(w401) -> ()
        n200 = Select(t=Aquire_State."Acquire" ("Acquire State"), s=w393, f=Aquire_State."WaitForWaveCompletion" ("Acquire State")) -> (s? t:f=w408:T3)
        n201 = case shown="False" w393 {
          tunnel: w395 -> [_ w411]
          tunnel: [u16 0 w411] -> w394
          frame False {
          }
          frame True {
          }
        }
      }
      frame "WaitForWaveCompletion" {
        n202 = Increment(x=w418) -> (x+1=w416:u16)
        n203 = Greater?(x=w412, y=w416) -> (0:w415:bool)
        n204 = Select(t=Aquire_State."WaitForWaveCompletion" ("Acquire State"), s=w415, f=Aquire_State."CheckAvg" ("Acquire State")) -> (s? t:f=w421:T3)
      }
      frame "CheckAvg" {
        n205 = Increment(x=w428) -> (x+1=w426:u16)
        n206 = Greater?(x=w427, y=w426) -> (0:w424:bool)
        n207 = Select(t=Aquire_State."AlignWave" ("Acquire State"), s=w424, f=Aquire_State."Idle") -> (s? t:f=w432:T3)
        n208 = xnode ("FIFO Method Node")("Element"=w424, "Timeout"=0) -> ()  [unwired: 1 in, 2 out]
      }
    }
  }
  n209 = while "Configuration Loop" {
    stop <- FALSE stop-if-true
    # "After the NI 5772 is powered on, the CLIP core provides the module with a default configuration. This loop updates the host VI to the status of the NI 5772 through the Initalization Done Signal. Additionally, this loop configures the Sample clock selection for the NI 5772. Refer to the Clock Select (Host).vi Host VI for more information about how this example configures the clock."
    n210 = xnode "FPGA I/O Node"("IO Module\\User Command"="User Command", "IO Module\\User Data 0"="User Data 0", "IO Module\\User Data 1"="User Data 1", "IO Module\\User Command Commit"="User Command Commit") -> ("IO Module\\User Command Idle"=→"User Command Idle":bool, "IO Module\\User Command Status"=→"User Command Status":u8, "IO Module\\PLL Locked"=→"PLL Locked":bool, "IO Module\\User Error"=w442:u8, "IO Module\\Initialization Done"=→"Configured?":bool)  [unwired: 9 in, 9 out]
    n211 = Not Equal To 0?(x=w442) -> (x != 0?=→"User Error":bool)
  }
  n212 = while "Data Validation/Calculation Loop" {
    stop <- FALSE stop-if-true
    n213 = Scale By Power Of 2(n="AvgCount_powerOf2", x=1 ("Timeout")) -> (x*2^n=w468:i32)
    n214 = To Unsigned Word Integer(number=w468) -> (unsigned 16bit integer=w465:u16)
    n215 = Multiply(x="Delay (us)", y=sgl 200.0) -> (x*y=w461:u16)
    n216 = Divide(x="WaveSampleCount", y="Wave Sampling Rate") -> (x/y=w452:sgl)
    n217 = In Range and Coerce(upper limit=u16 65535, x=w461, lower limit=u16 1) -> (coerced(x)=w453:u16)  [unwired: 1 out]
    "Delay after Trig [cycles]" <- w453
    n218 = In Range and Coerce(upper limit=u16 65535, x=w465, lower limit=u16 1) -> (coerced(x)=→"AvgCount":u16)  [unwired: 1 out]
    n219 = Multiply(x=w452, y=sgl 200000000.0) -> (x*y=w449:sgl)
    n220 = Add(x="Samples Per Trigger", y=w453) -> (x+y=w450:u16)
    n221 = Subtract(x=w449, y=w450) -> (x-y=→"WaitForWave\nCompletion":u16)
    n222 = call "Loop Timer"("Count(uSec)"=u32 100 ("Count(mSec)")) -> ()  [unwired: 1 out]
  }
  n223 = while "TrigOut Loop" {
    stop <- FALSE stop-if-true
    n224 = xnode ("FIFO Method Node")("Timeout"=0) -> ("Element"=w471:bool)  [unwired: 1 in, 2 out]
    n225 = case shown="True" w471 {
      frame False {
      }
      frame True {
        n226 = flat-sequence {
          frame #0 {
            n227 = xnode "FPGA I/O Node"("PXI_Trig1"=TRUE) -> ()  [unwired: 1 in, 1 out]
          }
          frame #1 {
            n228 = call "Wait"("Count(Ticks)"=u32 20 ("Count(uSec)")) -> ()  [unwired: 1 out]
          }
          frame #2 {
            n229 = xnode "FPGA I/O Node"("PXI_Trig1"=FALSE) -> ()  [unwired: 1 in, 1 out]
          }
        }
      }
    }
  }
  n230 = node-c288() -> (w11:T4)  [unwired: 1 in]
  n231 = timed-loop "Trigger In Loop" {
    timing: w11 -> [_]
    timing-out: [_] -> w10
    stop <- FALSE stop-if-true
    # "Triggering is handeled in the 40MHz Loop to remove the signal Jitter and false triggers"
    n232 = xnode "FPGA I/O Node"() -> ("IO Module\\Asynchronous Trigger Input"=w482:bool)  [unwired: 1 in, 1 out]
    n233 = call <instrlib>:"Detect Rising Edge.vi"("signal"=w482) -> ("edge detected"=w479:bool)  [unwired: 14 in]
    n234 = xnode ("FIFO Method Node")("Element"=w482, "Timeout"=0) -> ()  [unwired: 1 in, 2 out]
    n235 = call-poly <instrlib>:"Count Up.vi"("increment"=w479, "reset"="Clear Count") -> ("count out"=→"Trig Count":u64)  [unwired: 13 in]
  }
  n236 = node-c288(w10) -> ()
  n237 = node-c288(w6) -> ()
  n238 = node-c288(w15) -> ()
